vi "Write Lines.vi"(8 "error in (no error)":errorcluster, 10 "Lines":T1[](array[typedef]), 11 "OPC UA configuration in":refnum<class "OPC UA configuration.lvclass">) -> (0 "error out":errorcluster, 3 "OPC UA configuration out":refnum<class "OPC UA configuration.lvclass">)   [LabVIEW 2013, in "OPC UA configuration.lvclass"]
uses:
  OPC UA configuration.lvclass
  Line.ctl
  <vilib>/NI/Tag Bus Module Framework/channel/TBM channel.lvclass
  OPC UA configuration.lvclass/OPC UA configuration.ctl
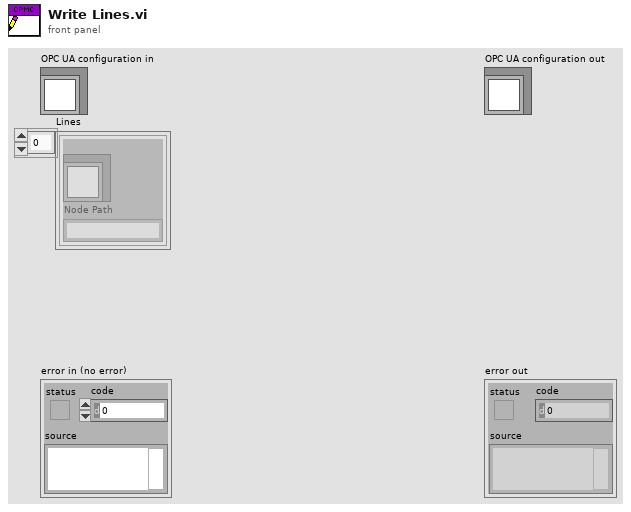
[diagram p1: front panel]
types:
  T1 = typedef "OPC UA configuration.lvclass/Line.ctl" = cluster{"channel":refnum<class "TBM channel.lvclass">, "Node Path":string}
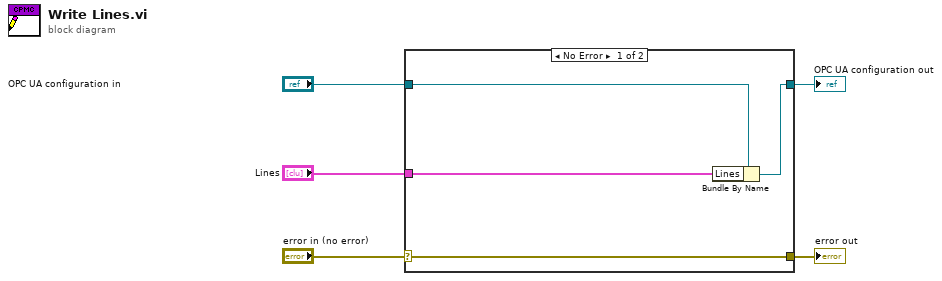
[diagram p0: block diagram]
diagram:
  n1 = case shown="No Error" "error in (no error)" {
    selector: "error in (no error)" -> [w9 w10]
    tunnel: [w9 w10] -> w4
    tunnel: [w7 w11] -> w2
    tunnel: "OPC UA configuration in" -> [w8 w11]
    tunnel: "Lines" -> [w6 _]
    frame No Error {
      n2 = Bundle By Name(cluster=w8, "Lines"=w6) -> (w7:refnum<class "OPC UA configuration.lvclass">)
    }
    frame Error {
    }
  }
  "error out" <- w4
  "OPC UA configuration out" <- w2
